vi "WriteVerify Mfg Serial Number.vi"(8 "error in":errorcluster, 11 "Serial Number":string) -> (0 "error out":errorcluster)   [LabVIEW 2015]
panel:
  out "Written Serial Number":string
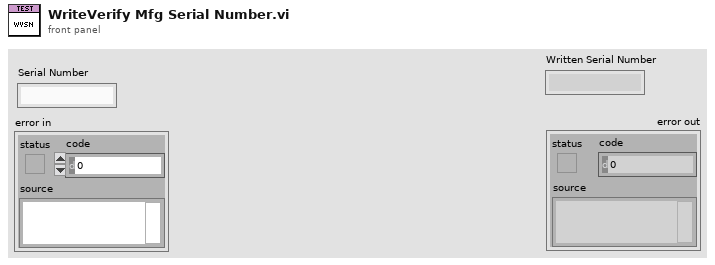
[diagram p1: front panel]
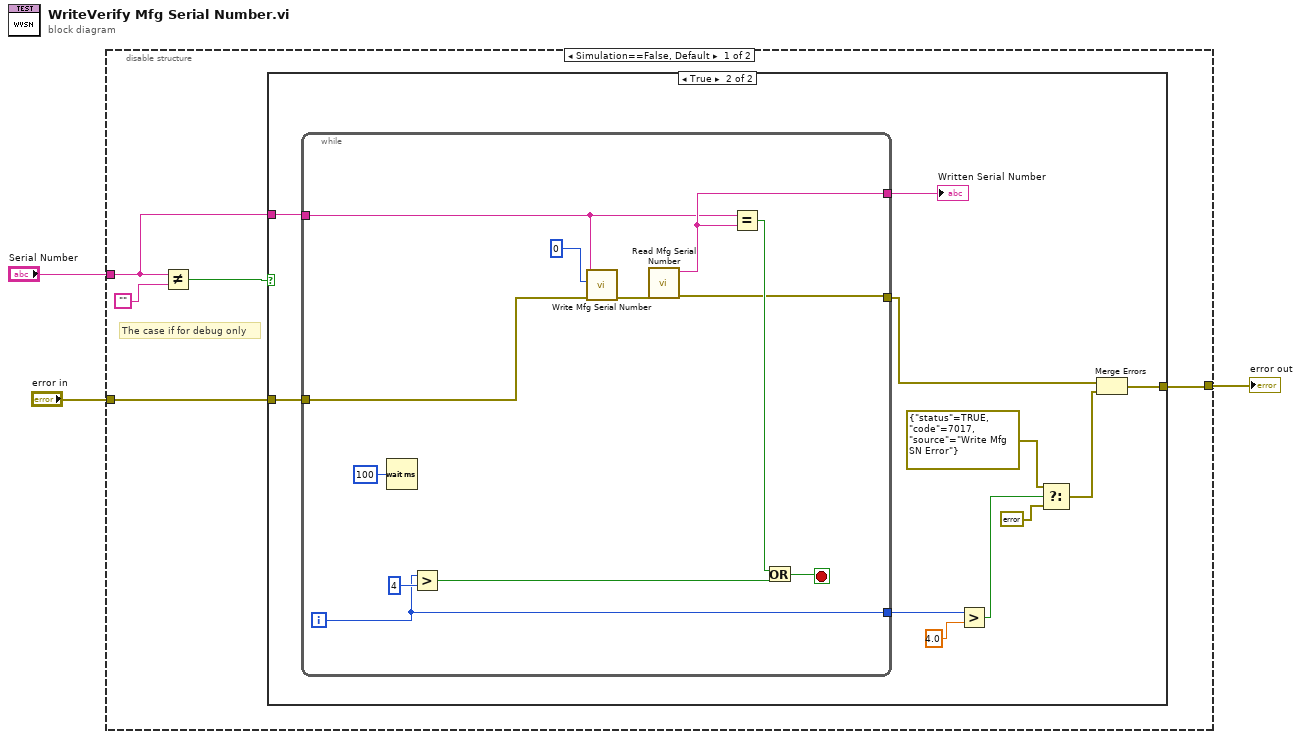
[diagram p0: block diagram]
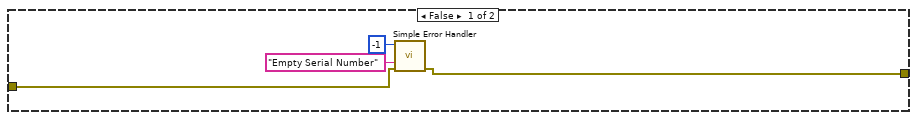
[diagram p2: hidden frame]
diagram:
  n1 = disable-structure shown="Simulation==False, Default" {
    disable-tunnel: "error in" -> [w8 w36]
    disable-tunnel: [w7 w36] -> w2
    disable-tunnel: "Serial Number" -> [w4 _]
    frame condition #0 (active) {
      # "The case if for debug only"
      n2 = Not Equal?(x=w4, y="") -> (x != y?=w5:bool)
      n3 = case shown="True" w5 {
        tunnel: w8 -> [w12 w23]
        tunnel: [w11 w15] -> w7
        tunnel: w4 -> [_ w13]
        frame False {
          n4 = call <vilib>:"Simple Error Handler.vi"("error code (no error:0)"=-1, "error source (\" \")"="Empty Serial Number" ("error source (\" \")"), "error in (no error)"=w12) -> ("error out"=w11:errorcluster)  [unwired: 2 in, 4 out]
        }
        frame True {
          n5 = while {
            tunnel: w23 -> [w29]
            tunnel: w13 -> [w26]
            tunnel: [w24] -> w16
            tunnel: [w31] -> w21
            tunnel: [w27] -> w14
            i -> [w31]
            stop <- w33 stop-if-true
            n6 = Wait (ms)(milliseconds to wait=u32 100) -> ()  [unwired: 1 out]
            n7 = Greater?(x=w31, y=4) -> (0:w34:bool)
            n8 = call "Write Mfg Serial Number.vi"("error in"=w29, "Start Address"=u8 0, "Serial Number"=w26) -> ("error out"=w28:errorcluster)  [unwired: 8 in]
            n9 = call "Read Mfg Serial Number.vi"("error in"=w28) -> ("error out"=w24:errorcluster, "Serial Number"=w27:string)  [unwired: 9 in]
            n10 = Equal?(x=w26, y=w27) -> (x = y?=w25:bool)
            n11 = Or(x=w25, y=w34) -> (x .or. y?=w33:bool)
          }
          "Written Serial Number" <- w14
          n12 = Greater?(x=w21, y=4.0) -> (0:w20:bool)
          n13 = Select(t=errorcluster {"status"=TRUE, "code"=7017, "source"="Write Mfg SN Error"} ("f"), s=w20, f=errorcluster {"status"=FALSE, "code"=0, "source"=""}) -> (s? t:f=w17:errorcluster)
          n14 = Merge Errors(w16, w17) -> (w15:errorcluster)
        }
      }
    }
    frame condition #1 {
    }
  }
  "error out" <- w2
